vi "Day 19-Brute Force.vi"() -> ()   [LabVIEW 2021]
uses:
  a026a2ab-26f8-4a39-8e1d-061d06921e16.vi
  ec2ad6d2-8c51-4d9e-985b-4ec09321e157.vi
  <vilib>/Utility/file.llb/Read Delimited Spreadsheet (string).vi
  <vilib>/Analysis/Matrix/Numeric/Conversions/Array To Matrix - RA.vi
  <vilib>/Analysis/Matrix/Numeric/Multiply/Multiply - RM,RM.vi
  <vilib>/Analysis/Matrix/Numeric/Conversions/Matrix To Array - RM.vi
  <vilib>/regexp/Match Regular Expression.xnode
  <vilib>/Analysis/Matrix/NI_Matrix.lvlib
panel:
  out "size":i32
  out "All Coordinates":i32[][][](array[numeric])
  out "Input":string[](array[string])
  in  "Input File":enum32{"example input", "input"}(radio)
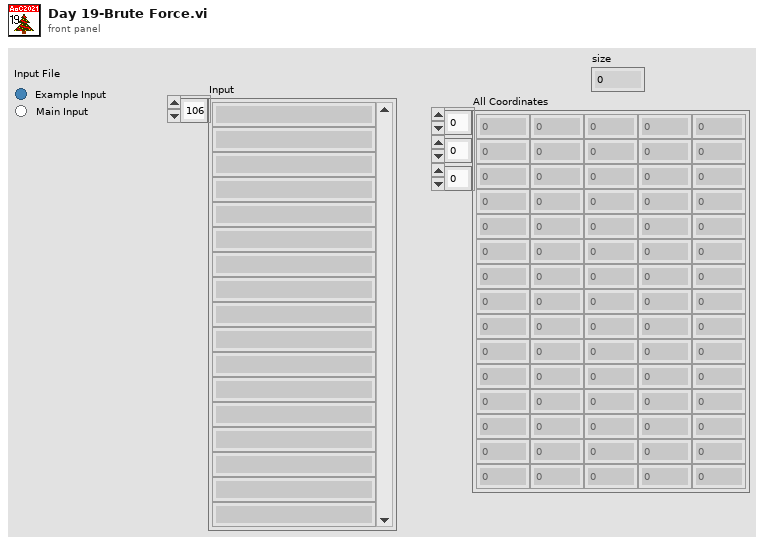
[diagram p1: front panel]
types:
  T1 = typedef "NI_Matrix.lvlib/RealMatrix.ctl" = dbl[][]
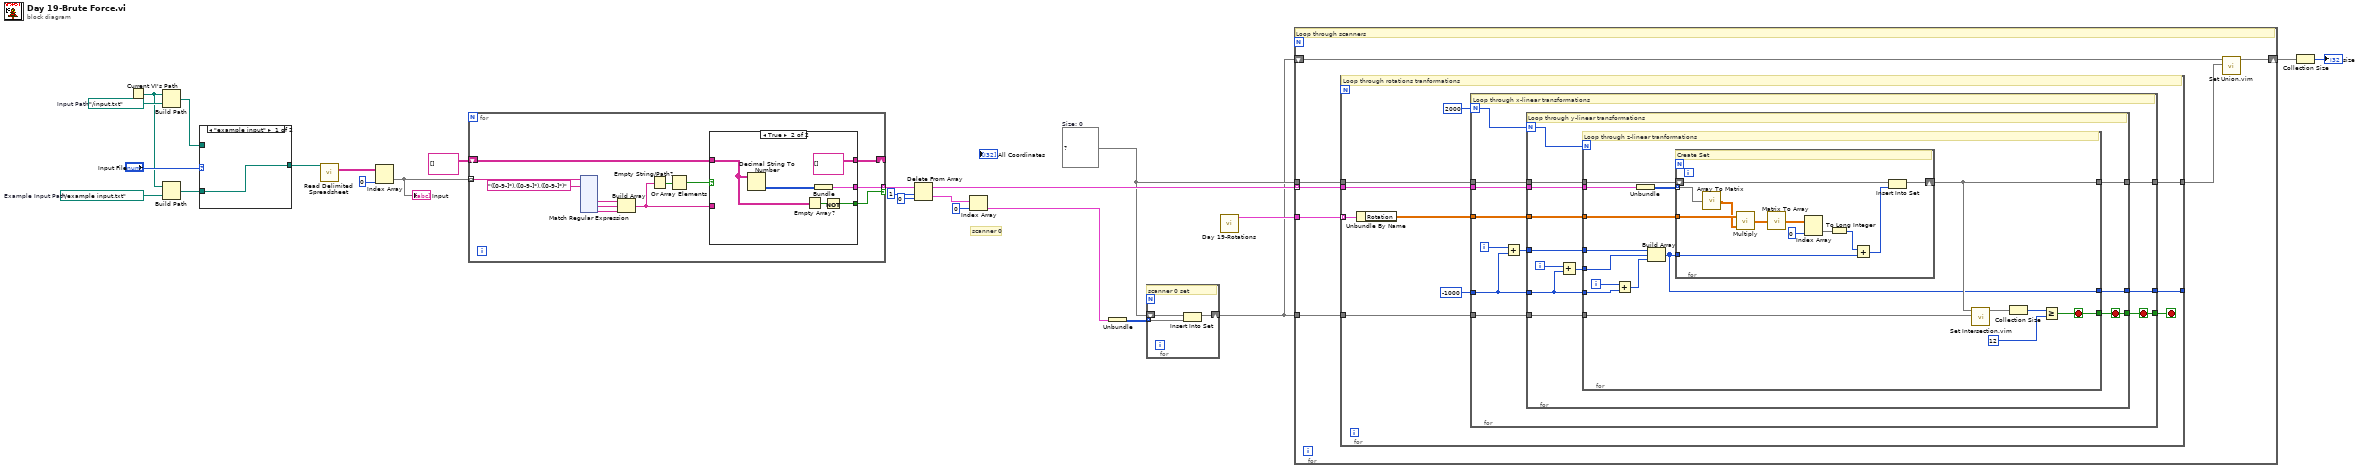
[diagram p0: block diagram]
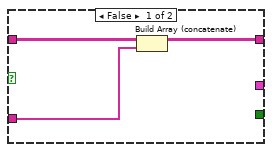
[diagram p2: hidden frame]
diagram:
  w9 = set{i32[]} {}  # Size: 0
  w23 = path "../example input.txt"  # Example Input Path
  w24 = path "../input.txt"  # Input Path
  # "scanner 0"
  n1 = Current VI's Path() -> (path=w18:path)
  n2 = Build Path(base path=w18, name or relative path=w24) -> (appended path=w21:path)
  n3 = Build Path(base path=w18, name or relative path=w23) -> (appended path=w20:path)
  n4 = case shown="\"example input\"" "Input File" {
    tunnel: w21 -> [_ w26]
    tunnel: w20 -> [w25 _]
    tunnel: [w25 w26] -> w19
    frame "example input" {
    }
    frame "input" {
    }
  }
  n5 = call-poly <vilib>:"Read Delimited Spreadsheet.vi"("file path (dialog if empty)"=w19) -> ("all rows"=w17:string[][])  [unwired: 9 in, 5 out]
  n6 = Index Array(array=w17, index (col)=0 ("disabled index (col)")) -> (element=w15:string[])  [unwired: 1 in]
  "Input" <- w15
  n7 = for {
    tunnel: w15 -> [w38] mode=indexing
    shift-right: [w32] -> _
    shift-left: string[][] [] -> [w33]
    tunnel: [w31] -> w3 mode=indexing if=w30
    n8 = xnode "Match Regular Expression"("input string"=w38, "regular expression"="([0-9-]*),([0-9-]*),([0-9-]*)") -> ("submatch 1"=w36:string, "submatch 2"=w35:string, "submatch 3"=w34:string)  [unwired: 4 in, 5 out]
    n9 = Build Array(w36, w35, w34) -> (w29:string[])
    n10 = Empty String/Path?(string/path=w29) -> (empty?=w28:bool[])
    n11 = Or Array Elements(Boolean array=w28) -> (logical OR=w27:bool)
    n12 = case shown="True" w27 {
      tunnel: w29 -> [w41 _]
      tunnel: w33 -> [w40 w42]
      tunnel: [w39 string[][] []] -> w32
      tunnel: [_ w44] -> w31
      tunnel: [_ w45] -> w30
      frame False {
        n13 = Build Array (concatenate)(w40, w41) -> (w39:string[][])
      }
      frame True {
        n14 = Decimal String To Number(string=w42) -> (number=w43:i32[][])  [unwired: 2 in, 1 out]
        n15 = Empty Array?(array=w42) -> (empty?=w46:bool)
        n16 = Bundle(w43) -> (w44:cluster{i32[][]})  [unwired: 1 in]
        n17 = Not(x=w46) -> (.not. x?=w45:bool)
      }
    }
  }
  n18 = Delete From Array(array=w3, length=1, index=0 ("index (page)")) -> (deleted portion=w8:cluster{i32[][]}[], array with subset deleted=w11:cluster{i32[][]}[])
  n19 = Index Array(array=w8, index=0 ("index (page)")) -> (element=w2:cluster{i32[][]})
  n20 = Unbundle(w2) -> (w1:i32[][])
  n21 = for {
    tunnel: w1 -> [w169] mode=indexing
    shift-right: [w171] -> w6
    shift-left: w9 -> [w170]
    # "scanner 0 set"
    n22 = Insert Into Set(10:w169, 11:w170) -> (3:w171:set{i32[]})  [unwired: 1 out]
  }
  n23 = call "Day 19-Rotations.vi"() -> ("Rotations"=w7:cluster{"Rotation":T1}[])  [unwired: 11 in]
  n24 = for {
    tunnel: w11 -> [w177] mode=indexing
    tunnel: w6 -> [w172]
    tunnel: w9 -> [w178]
    tunnel: w7 -> [w176]
    shift-right: [w174] -> w5
    shift-left: w6 -> [w173]
    # "Loop through scanners"
    n25 = for {
      tunnel: w178 -> [w188]
      tunnel: w172 -> [w187]
      tunnel: w177 -> [w186]
      tunnel: w176 -> [w185] mode=indexing
      tunnel: [w181] -> w175
      tunnel: [w180] -> _
      stop <- w179 stop-if-true
      # "Loop through rotations tranformations"
      n26 = Unbundle By Name(w185) -> ("Rotation"=w184:T1)
      n27 = for {
        N: 2000 -> [w195]
        tunnel: w188 -> [w199]
        tunnel: w186 -> [w198]
        tunnel: w184 -> [w197]
        tunnel: w187 -> [w196]
        tunnel: -1000 -> [w192]
        tunnel: [w191] -> w180
        tunnel: [w190] -> w181
        tunnel: [w189] -> w179
        i -> [w194]
        stop <- w189 stop-if-true
        # "Loop through x-linear transformations"
        n28 = Add(x=w194, y=w192) -> (x+y=w193:i32)
        n29 = for {
          N: w195 -> [w207]
          tunnel: w199 -> [w211]
          tunnel: w198 -> [w210]
          tunnel: w197 -> [w209]
          tunnel: w196 -> [w208]
          tunnel: w193 -> [w205]
          tunnel: w192 -> [w203]
          tunnel: [w202] -> w191
          tunnel: [w201] -> w190
          tunnel: [w200] -> w189
          i -> [w206]
          stop <- w200 stop-if-true
          # "Loop through y-linear transformations"
          n30 = Add(x=w206, y=w203) -> (x+y=w204:i32)
          n31 = for {
            N: w207 -> [_]
            tunnel: w211 -> [w227]
            tunnel: w210 -> [w216]
            tunnel: w209 -> [w226]
            tunnel: w208 -> [w217]
            tunnel: w205 -> [w223]
            tunnel: w204 -> [w222]
            tunnel: w203 -> [w224]
            tunnel: [w212] -> w202
            tunnel: [w213] -> w201
            tunnel: [w214] -> w200
            i -> [w225]
            stop <- w214 stop-if-true
            # "Loop through z-linear tranformations"
            n32 = Add(x=w225, y=w224) -> (x+y=w221:i32)
            n33 = Unbundle(w216) -> (w215:i32[][])
            n34 = Build Array(w223, w222, w221) -> (w212:i32[])
            n35 = for {
              tunnel: w215 -> [w238] mode=indexing
              tunnel: w226 -> [w237]
              tunnel: w212 -> [w231]
              shift-right: [w228] -> w213
              shift-left: w227 -> [w239]
              # "Create Set"
              n36 = call-poly <vilib>:"Array To Matrix.vi"("Real 1D Array"=w238) -> ("Real Matrix (Column Vector)"=w236:T1)
              n37 = call-poly <vilib>:"Multiply.vi"("Real Matrix B"=w236, "Real Matrix A"=w237) -> ("A * B"=w235:T1)
              n38 = call-poly <vilib>:"Matrix To Array.vi"("Real Matrix"=w235) -> ("Real 2D Array"=w234:dbl[][])
              n39 = Index Array(array=w234, index (col)=0 ("disabled index (col)")) -> (element=w232:dbl[])  [unwired: 1 in]
              n40 = To Long Integer(number=w232) -> (32bit integer=w230:i32[])
              n41 = Add(x=w230, y=w231) -> (x+y=w229:i32[])
              n42 = Insert Into Set(10:w229, 11:w239) -> (3:w228:set{i32[]})  [unwired: 1 out]
            }
            n43 = call "Set Intersection.vim"("set 2"=w217, "set 1"=w213) -> ("intersection"=w220:set{i32[]})  [unwired: 9 in]
            n44 = Collection Size(1:w220) -> (0:w219:i32)
            n45 = Greater Or Equal?(x=w219, y=12) -> (x >= y?=w214:bool)
          }
        }
      }
    }
    n46 = call "Set Union.vim"("set 2"=w175, "set 1"=w173) -> ("union"=w174:set{i32[]})  [unwired: 9 in]
  }
  n47 = Collection Size(1:w5) -> (0:→"size":i32)
